vi "SectionA04_Week2_Stus.vi"() -> ()   [LabVIEW 2013]
panel:
  out "X<Y":bool
  out "X=Y":bool
  out "X>Y":bool
  out "sin(X)":dbl
  out "2^X - ln(Y)":dbl
  out "sqrt(X/Y) + 1":dbl
  out "1/(X*Y)":dbl
  out "abs(X-Y)":dbl
  out "X+Y":dbl
  in  "Y":dbl
  in  "X":dbl
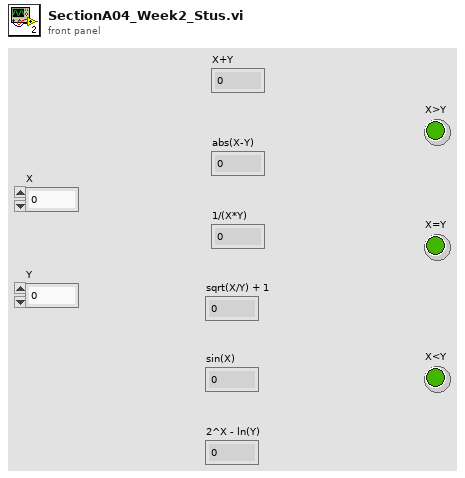
[diagram p1: front panel]
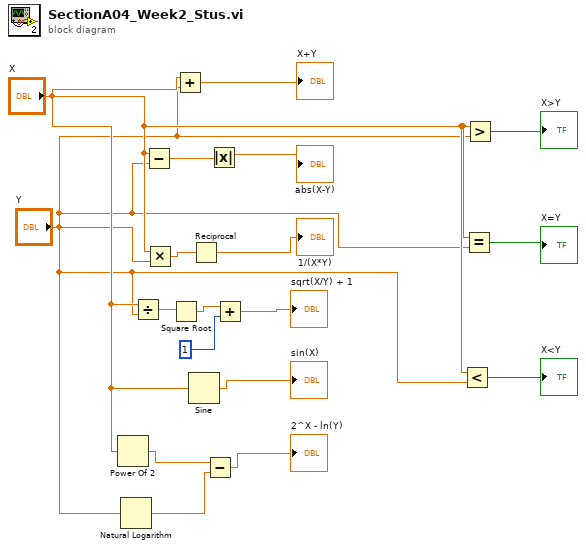
[diagram p0: block diagram]
diagram:
  n1 = Power Of 2(x="X") -> (2^x=w9:dbl)
  n2 = Natural Logarithm(1:"Y") -> (0:w8:dbl)
  n3 = Divide(x="X", y="Y") -> (x/y=w13:dbl)
  n4 = Subtract(x="X", y="Y") -> (x-y=w17:dbl)
  n5 = Multiply(x="X", y="Y") -> (x*y=w15:dbl)
  n6 = Square Root(x=w13) -> (sqrt(x)=w12:dbl)
  n7 = Add(x="X", y="Y") -> (x+y=→"X+Y":dbl)
  n8 = Sine(x="X") -> (sin(x)=→"sin(X)":dbl)
  n9 = Reciprocal(x=w15) -> (1/x=→"1/(X*Y)":dbl)
  n10 = Subtract(x=w9, y=w8) -> (x-y=→"2^X - ln(Y)":dbl)
  n11 = Absolute Value(x=w17) -> (abs(x)=→"abs(X-Y)":dbl)
  n12 = Add(x=w12, y=1) -> (x+y=→"sqrt(X/Y) + 1":dbl)
  n13 = Less?(x="X", y="Y") -> (x < y?=→"X<Y":bool)
  n14 = Equal?(x="X", y="Y") -> (x = y?=→"X=Y":bool)
  n15 = Greater?(x="X", y="Y") -> (0:→"X>Y":bool)
